vi "DHE_SetExtShutter.vi"(2 "Ext_Shutter":bool) -> ()   [LabVIEW 2016]
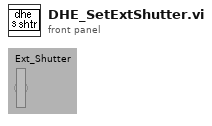
[diagram p1: front panel]
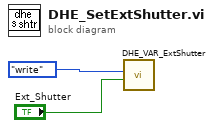
[diagram p0: block diagram]
diagram:
  n1 = call "DHE_VAR_ExtShutter.vi"("ext. shutter"="Ext_Shutter", "action"=enum16{"read", "write"}."write") -> ()  [unwired: 10 out]
